vi "UITimeoutStep.vi"(8 "error in (no error)":errorcluster, 11 "RealWorkActor in":refnum<class "RealWorkActor.lvclass">) -> (0 "error out":errorcluster, 3 "RealWorkActor out":refnum<class "RealWorkActor.lvclass">)   [LabVIEW 2021, in "RealWorkActor.lvclass"]
uses:
  RealWorkActor.lvclass
  RealWorkActor.lvclass/RealWorkActor.ctl
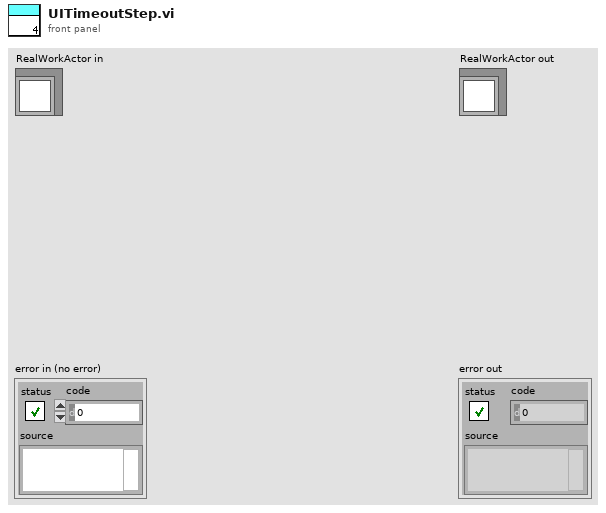
[diagram p1: front panel]
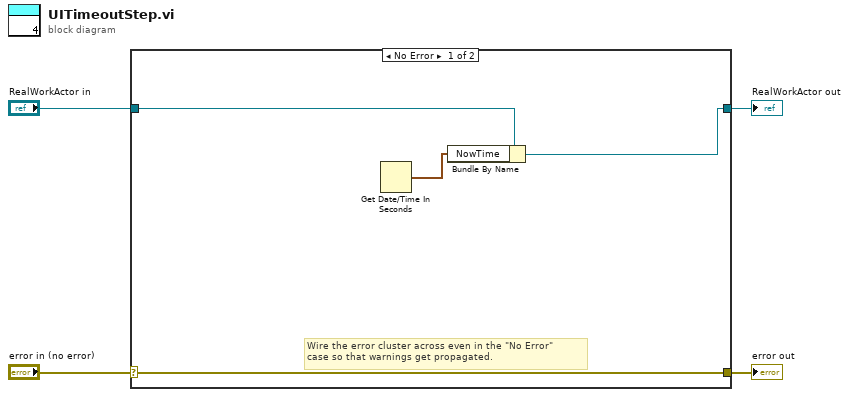
[diagram p0: block diagram]
diagram:
  n1 = case shown="No Error" "error in (no error)" {
    selector: "error in (no error)" -> [w8 w10]
    tunnel: [w8 w10] -> w3
    tunnel: [w5 w9] -> w1
    tunnel: "RealWorkActor in" -> [w6 w9]
    frame No Error {
      # "Wire the error cluster across even in the \"No Error\"\ncase so that warnings get propagated."
      n2 = Get Date/Time In Seconds() -> (seconds since 1Jan1904=w7:timestamp)
      n3 = Bundle By Name(cluster=w6, "NowTime"=w7) -> (w5:refnum<class "RealWorkActor.lvclass">)
    }
    frame Error {
    }
  }
  "error out" <- w3
  "RealWorkActor out" <- w1
